vi "2 Channel Oscilloscope-iterate_filename.vi"() -> ()   [LabVIEW 2013]
doc: "The Two Channel Oscilloscope acquires and displays waveforms from one or two channels. Enter your Channel(s) and run the VI. While running, you can adjust the vertical position and volts per division, as well as the timebase. The Polarity can be set to get the best use of the range of your DAQ device. This VI supports digital and analog triggering. For digital triggering, you must connect the appropriate high-to-low or low-to-high TTL trigger signal to the trigger pin of your DAQ device. For analog trigger you set the trigger Level and Slope. View the help window description of each control for more information about its use."
panel:
  in  "input terminal configuration":i32(ring)=-1 items=["default"=-1, "RSE"=10083, "NRSE"=10078, "Differential"=10106, "Pseudodifferential"=12529]
  out "File Name Out Location":path caption="File Name Out"
  in  "Save to File":bool
  in  "digital source":tag="/Dev1/PFI0"
  in  "Trigger not recieved":string="Trigger Level is Out of Range or Trigger was not Recieved"
  in  "Channel B":tag="Dev1/ai1"
  in  "Channel A":tag="Dev1/ai0"
  in  "trigger support":string="Your hardware does not support this trigger mode."
  in  "invalid timebase":string="Invalid Timebase"
  out "Acquired":bool=TRUE
  in  "A/B switches":T1={"Position A"=-0.7490503006368473, "on/off A"=TRUE, "Position B"=-0.4188678921837484, "on/off B"=TRUE} {"Position B" min=-5.0 max=5.0 scale=-5.0..5.0 scale format="%0.1f"; "Position A" min=-5.0 max=5.0 scale=-5.0..5.0 scale format="%0.1f"}
  in  "Stop":bool
  in  "Timebase":u32(knob)=7 scale=0.0..11.0
  in  "Acquire On":bool=TRUE
  in  "Acquire Once":bool
  out "Timeout":bool
  in  "Slope":bool
  in  "Volts/Div B":u32(knob)=6 scale=0.0..9.0
  in  "Mode":u16(ring) items=["None", "Digital", "Hardware  Analog ", "Reference Analog"]
  in  "Position":i32(knob) min=0 max=497 scale=0.0..497.0
  in  "Level":dbl(knob)=0.5 min=-10.0 max=10.0 step=0.1 scale=-10.0..10.0
  in  "Channel":bool
  in  "Volts/Div A":u32(knob)=6 scale=0.0..9.0
  out "scope graph":sgl[][](graph)=[[-0.2881528, -0.23340708, -0.1802715, -0.12874603, -0.080118895, -0.032135844, 0.014237046, 0.054813385, 0.093135476, 0.12759316, 0.15850842, 0.182661, 0.2039153, 0.22001702, 0.23289835, 0.24320346, 0.24867809, 0.2538306, 0.2551188, 0.2586611, 0.25801712, 0.25544077, 0.25254244, 0.24738991, 0.23805094, 0.22420347, 0.2077797, 0.18813556, 0.16011858, 0.12888128, 0.093779504, 0.054169297, 0.011982858, -0.032779932, -0.081729114, -0.13228846, -0.18284774, -0.2366274, -0.2916952, -0.3451528, -0.40215275, -0.45689845, -0.5122882, -0.56864405, -0.6214576, -0.67620325, -0.72772855, -0.7821522, -0.83206725, -0.87844, -0.9248128, -0.96796525, -1.0091854, -1.043643, -1.0764903, -1.1070834, -1.1305919, -1.1476595, -1.162151, -1.1734221, -1.1850153, -1.1885576, -1.1917781, -1.1940322, -1.1972525, -1.1991848, -1.1943543, -1.1888797, -1.1834052, -1.1740662, -1.1573205, -1.1389647, -1.1164224, -1.0900156, -1.0545921, -1.0194905, -0.9795584, -0.936084, -0.8903552, -0.839152, -0.7895589, -0.7399658, -0.6852201, -0.6304745, -0.5754068, -0.519695, -0.46527132, -0.4076273, -0.3528816, -0.29749182, -0.24467826, -0.19057655, -0.13905114, -0.089135885, -0.04083079, 0.0026438236, 0.048050642, 0.08637273, 0.12018633, 0.15110165, 0.17879659, 0.1994068, 0.21615261, 0.22838992, 0.23837298, 0.24771196, 0.25157636, 0.25318652, 0.25576288, 0.25769502, 0.25737303, 0.25189847, 0.2461018, 0.23644078, 0.22549158, 0.20874578, 0.18716949, 0.16301692, 0.13338977, 0.09893209, 0.05835575, 0.017457426, -0.027627349, -0.0759325, -0.12649184, -0.17801726, -0.22922063, -0.28525454, -0.34257653, -0.39700022, -0.45013577, -0.50745773, -0.5641356, -0.6198474, -0.6749151, -0.7267624, -0.7789318, -0.83077914, -0.8797282, -0.92513484, -0.9695754, -1.0120838, -1.0484735, -1.0800326, -1.1093377, -1.1351002, -1.1560323, -1.1734221, -1.1834052, -1.1921, -1.201117, -1.2046593, -1.2053034, -1.2085238, -1.2101339, -1.2085238, -1.2024051, -1.1943543, -1.1859814, -1.1750324, -1.1550663, -1.132846, -1.1057953, -1.0745581, -1.0391345, -0.99855834, -0.95605, -0.9122535, -0.86298245, -0.8127453, -0.75799966, -0.7067964, -0.6530168, -0.596983, -0.5406272, -0.48427132, -0.43049172, -0.37574598, -0.31874603, -0.26367825, -0.21054268, -0.15901726, -0.10684776, -0.058220625, -0.014423966, 0.030982852, 0.071881175, 0.10794902, 0.14015245, 0.16784745, 0.19006783, 0.20745766, 0.22420347, 0.23225433, 0.24094927, 0.24738991, 0.24867809, 0.25125438, 0.26188153, 0.25415272, 0.25093234, 0.24481368, 0.23579669, 0.22645772, 0.21164411, 0.19167799, 0.16688132, 0.13822025, 0.10505074, 0.06801677, 0.02518624, -0.020220578, -0.067237556, -0.116830826, -0.16835624, -0.22181386, -0.27527148, -0.32937315, -0.385407, -0.4420849, -0.49876282, -0.55222034, -0.6072881, -0.66396594, -0.7180675, -0.7689488, -0.82079613, -0.86974514, -0.91869414, -0.9618466, -1.0027448, -1.0426768, -1.0774564, -1.1077275, -1.1318799, -1.1534561, -1.1695578, -1.1843712, -1.191134, -1.2001508, -1.2065915, -1.2088457, -1.2078797, -1.2082016, -1.2078797, -1.2062695, -1.2007949, -1.1895238, -1.1769645, -1.1615069, -1.1396087, -1.1122359, -1.0826089, -1.0491176, -1.0104735, -0.96667707, -0.92030436, -0.8726435, -0.8256266, -0.77313524, -0.71903366, -0.66396594, -0.6108304, -0.5535085, -0.49876282, -0.44240695, -0.38701716, -0.33227146, -0.27752572, -0.22245795, -0.1699664, -0.12101722, -0.06916976, -0.022474825, 0.01938963, 0.060609996, 0.09732193, 0.1321016, 0.16011858, 0.182661, 0.20262712, 0.21840686, 0.2312882, 0.2377289, 0.24449164, 0.24738991, 0.25125438, 0.25286454, 0.25318652, 0.2499662, 0.24642384, 0.23869503, 0.22838992, 0.21357632, 0.19683051, 0.17235589, 0.14466095, 0.111813426, 0.07703376, 0.03581339, -0.007983267, -0.055966377, -0.10394943, -0.15450877, -0.20539016, -0.26239014, -0.31649178, -0.3709155, -0.42694935, -0.48427132, -0.53966105, -0.59408474, -0.64947444, -0.70260996, -0.75799966, -0.80952495, -0.85718584, -0.9042027, -0.9525076, -0.99469393, -1.0323718, -1.0671513, -1.1006428, -1.1273715, -1.1489477, -1.1647272, -1.1798629, -1.1921, -1.1988628, -1.2024051, -1.2059474, -1.2130322, -1.210778, -1.2082016, -1.2078797, -1.2030492, -1.1959645, -1.181795, -1.1634392, -1.1457274, -1.122219, -1.0909817, -1.0558802, -1.0188464, -0.97988045, -0.93447375, -0.88552475, -0.83593166, -0.78569454, -0.73288107, -0.6778134, -0.62177956, -0.56864405, -0.5116441, -0.4552883, -0.39893243, -0.3441867, -0.29040706, -0.2346952, -0.18155962, -0.13035625, -0.081729114, -0.032779932, 0.011982858, 0.054169297, 0.0899151, 0.12437278, 0.15367794, 0.17944068, 0.19876271, 0.21583056, 0.22774583, 0.2370848, 0.24320346, 0.24706793, 0.25028825, 0.25189847, 0.25222045, 0.25028825, 0.24738991, 0.24030519, 0.23096615, 0.21776277, 0.1994068, 0.17879659, 0.15238976, 0.1195423, 0.08444053, 0.044830322, 0.0010336637, -0.045017183, -0.09461045, -0.14388168, -0.19637316, -0.24983081, -0.3061867, -0.36028838, -0.41374597, -0.471712, -0.52838993, -0.5824915, -0.6391694, -0.6913388, -0.74640644, -0.7982538, -0.84913504, -0.8955078, -0.94091445, -0.9863211, -1.025287, -1.0591005, -1.0916258, -1.1206088, -1.1454053, -1.1653713, -1.1769645, -1.1888797, -1.1991848, -1.2043374, -1.2069136, -1.2075577, -1.2127101, -1.2127101, -1.2072356, -1.201439, -1.1927441, -1.1850153, -1.1698798, -1.1492697, -1.1254393, -1.0987105, -1.0658633, -1.0256091, -0.985033, -0.94284666, -0.8967959, -0.8455927, -0.7953555, -0.7425421, -0.6903727, -0.6340169, -0.5786271, -0.52323735, -0.46881372, -0.41181377, -0.3548138, -0.29974604, -0.2475766, -0.1928308, -0.1406613, -0.090424, -0.04405111, 0.0019997954, 0.046762526, 0.08444053, 0.11922026, 0.14916945, 0.1762203, 0.19811869, 0.21389836, 0.22710174, 0.2370848, 0.24481368, 0.24835604, 0.25093234, 0.2544747, 0.25576288, 0.25479668, 0.25157636, 0.24384755, 0.23547465, 0.22388142, 0.2077797, 0.18620336, 0.16108471, 0.13145757, 0.09571171, 0.056423545, 0.01455909, -0.028915524, -0.07883078, -0.12681383, -0.18188167, -0.23437315, -0.2887969, -0.34354264, -0.40022054, -0.45657644, -0.5110001, -0.5657458, -0.62242365, -0.67652524, -0.7293387, -0.7815081, -0.83206725, -0.8826265, -0.926745, -0.97118556, -1.0107956, -1.0500836, -1.0813208, -1.1109478, -1.1331681, -1.1569985, -1.1737442, -1.1824391, -1.191456, -1.1988628, -1.2036933, -1.2040153, -1.2053034, -1.2056254, -1.2053034, -1.200473, -1.1908119, -1.182117, -1.1695578, -1.152168, -1.1280155, -1.0996766, -1.0700496, -1.034626, -0.99179566, -0.94896525, -0.9035586, -0.8565418, -0.8053385, -0.75220305, -0.6984235, -0.645288, -0.5905423, -0.53193223, -0.4765425, -0.42340696, -0.366085, -0.31037316, -0.25466132, -0.20023757, -0.15128845, -0.09911895, -0.049847722, -0.0047629476, 0.03742355, 0.07896596, 0.11406767, 0.14562708, 0.17074573, 0.19586444, 0.21389836, 0.22710174, 0.23805094, 0.2441696, 0.25157636, 0.25350863, 0.25640684, 0.25769502, 0.2551188, 0.25318652, 0.24900013, 0.23869503, 0.22838992, 0.21357632, 0.19264406, 0.16816944, 0.13822025, 0.10569477, 0.067050695, 0.026152313, -0.019254506, -0.06498331, -0.11522061, -0.16771215, -0.22084779, -0.27559352, -0.32969517, -0.38572904, -0.4420849, -0.4977967, -0.55189836, -0.6076101, -0.66203374, -0.7183896, -0.76927084, -0.81983, -0.8691011, -0.91643995, -0.96281266, -1.0021007, -1.0394565, -1.0748801, -1.1057953, -1.1305919, -1.1508799, -1.1669815, -1.1830832, -1.1908119, -1.1969305, -1.201117, -1.2069136, -1.2088457, -1.2056254, -1.2056254, -1.2043374, -1.1966085, -1.1875916, -1.1727781, -1.1576426, -1.1370325, -1.1090156, -1.0771344, -1.0429989, -1.0062871, -0.9637788, -0.9180501, -0.86974514, -0.819186, -0.76862675, -0.71452516, -0.6607456, -0.6072881, -0.5525424, -0.4945764, -0.43822053, -0.38025448, -0.3271189, -0.27301723, -0.21794945, -0.16577995, -0.114254534, -0.06530535, -0.019898534, 0.024542153, 0.06479645, 0.101186335, 0.1340338, 0.16140676, 0.18684745, 0.2039153, 0.21679664, 0.23193228, 0.23837298, 0.24481368, 0.248034, 0.25028825, 0.25189847, 0.25189847, 0.24835604, 0.24577975, 0.23611873, 0.22581363, 0.21003395, 0.19264406, 0.16849148, 0.13983041, 0.10827106, 0.070271015, 0.030982852, -0.012491763, -0.06015283, -0.11006808, -0.16062742, -0.213763, -0.26722065, -0.32357654, -0.37800023, -0.43339002, -0.4897459, -0.54545766, -0.6027796, -0.65655917, -0.71066076, -0.7650844, -0.8166097, -0.8639486, -0.9116094, -0.9583042, -1.0001686, -1.0375243, -1.072948, -1.103219, -1.1322019, -1.1534561, -1.1695578, -1.1840492, -1.1953204, -1.2053034, -1.2069136, -1.2111, -1.2146423, -1.2143203, -1.2123882, -1.2082016, -1.2020831, -1.1978967, -1.1837273, -1.1673036, -1.1450833, -1.122863, -1.092592, -1.0581344, -1.0191684, -0.97730416, -0.9328636, -0.8845587, -0.83593166, -0.78247416, -0.732559, -0.6771693, -0.6208135, -0.5657458, -0.51132214, -0.45593235, -0.39700022, -0.34193245, -0.28750876, -0.23340708, -0.1802715, -0.12906808, -0.08044094, -0.033746004, 0.010694683, 0.054169297, 0.091525316, 0.12533891, 0.1533559, 0.17847455, 0.19844067, 0.21325427, 0.22613567, 0.23418653, 0.2415933, 0.2441696, 0.24771196, 0.24932212, 0.24900013, 0.24674588, 0.24288148, 0.2370848, 0.22613567, 0.21357632, 0.19457626, 0.17299998, 0.14627111, 0.115033805, 0.078321874, 0.038389623, -0.0037968159, -0.04952568, -0.09815282, -0.15257657, -0.20216978, -0.25594944, -0.3100511, -0.3683392, -0.42308494, -0.4765425, -0.53354245, -0.5898983, -0.645288, -0.69681334, -0.7505929, -0.80276227, -0.85428756, -0.90066034, -0.9454229, -0.9888973, -1.0291514, -1.0661852, -1.0967784, -1.1238291, -1.1479816, -1.1676255, -1.1792188, -1.191134, -1.201761, -1.2072356, -1.2075577, -1.2123882, -1.2352524, -1.2143203, -1.210778, -1.2046593, -1.1946763, -1.1869476, -1.1705239, -1.1508799, -1.1260834, -1.0990326, -1.0652192, -1.0256091, -0.985355, -0.9399483, -0.8955078, -0.8462367, -0.79310125, -0.7406099, -0.68876255, -0.6327287, -0.57572883, -0.520017, -0.4649493, -0.40859342, -0.35159346, -0.29716977, -0.24403417, -0.19057655, -0.1387291, -0.08784777, -0.0382545, 0.005542159, 0.04708457, 0.08540666, 0.121474504, 0.15013552, 0.17654234, 0.20005089, 0.21486443, 0.22742379, 0.23805094, 0.24577975, 0.24932212, 0.25254244, 0.2538306, 0.2538306, 0.25125438, 0.24900013, 0.24288148, 0.23354244, 0.22259331, 0.20552546, 0.18201697, 0.15786433, 0.12823719, 0.092169344, 0.052237093, 0.0097286105, -0.035678208, -0.08462739, -0.13293248, -0.18703419, -0.23984778, -0.29330537, -0.3480511, -0.404729, -0.46237305, -0.51550853, -0.57250845, -0.6272541, -0.68360996, -0.73545736, -0.7866606, -0.83721983, -0.8868129, -0.9335077, -0.97537196, -1.0165921, -1.05427, -1.0871174, -1.1132021, -1.1386427, -1.1573205, -1.1753544, -1.1869476, -1.1937102, -1.2001508, -1.2053034, -1.2085238, -1.2091677, -1.2088457, -1.2098119, -1.2049813, -1.1949984, -1.1843712, -1.1708459, -1.1541002, -1.1280155, -1.1012869, -1.0690836, -1.0349481, -0.995016, -0.94960934, -0.9022705, -0.8546096, -0.8046945, -0.751881, -0.6984235, -0.6443219, -0.5905423, -0.53193223, -0.4775086, -0.42018664, -0.3683392, -0.31101722, -0.25498334, -0.20184779, -0.15000027, -0.10008502, -0.050813794, -0.0054070354, 0.03581339, 0.076711714, 0.112457514, 0.14305079, 0.17138982, 0.19200003, 0.21003395, 0.22291529, 0.23386449, 0.23998314, 0.24545771, 0.24932212, 0.25093234, 0.25350863, 0.25093234, 0.248034, 0.2441696, 0.23547465, 0.22259331, 0.20713562, 0.18813556, 0.16237283, 0.13145757, 0.099576116, 0.06093204, 0.018101454, -0.027949393, -0.07496637, -0.1242376, -0.17544097, -0.22954267, -0.28428844, -0.33774602, -0.39281377, -0.45077983, -0.5071357, -0.56381357, -0.615983, -0.6720168, -0.72579634, -0.7798979, -0.8275588, -0.87682986, -0.9248128, -0.9698974, -1.0101515, -1.0465412, -1.0787445, -1.1122359, -1.1370325, -1.1553884, -1.172134, -1.1872696, -1.1978967, -1.2027271, -1.2062695, -1.2117441, -1.2133542, -1.2091677, -1.2111, -1.2065915, -1.1998289, -1.1901679, -1.1769645, -1.1592528, -1.1367104, -1.1112698, -1.0784225, -1.0423548, -1.004999, -0.96410084, -0.91515183, -0.86684686, -0.81725377, -0.7670166, -0.71194893, -0.6575253, -0.6027796, -0.549, -0.4929662, -0.43435612, -0.37896633, -0.3242206, -0.26915282, -0.21472913, -0.16288167, -0.11296642, -0.064017236, -0.015068054, 0.0267964, 0.06737274, 0.10344058, 0.13725418, 0.16527116, 0.18684745, 0.20455933, 0.21969497, 0.23289835, 0.23933905, 0.24481368, 0.24738991], [-0.12800416, -0.1273601, -0.12703806, -0.12800416, -0.12800416, -0.126394, -0.12671602, -0.12703806, -0.12703806, -0.12607196, -0.12574992, -0.126394, -0.12671602, -0.1273601, -0.12607196, -0.1254279, -0.126394, -0.126394, -0.1254279, 1.4750845, 4.1615305, 4.1624966, 4.1541233, 4.1557336, 4.157022, 4.1615305, 4.153157, 4.1544456, 4.156378, 4.1605644, 4.1618524, 4.1541233, 4.15509, 4.160242, 4.1612086, 4.1538014, 4.1554117, 4.157022, 4.1618524, 4.1457505, 4.1541233, 4.157022, 4.1628184, 4.164107, 4.1554117, 4.1576657, 4.164107, 4.164107, 4.1557336, 4.15831, 4.1673274, 4.166361, 4.1518693, 4.160242, 4.1618524, 4.1676493, 4.1699038, 4.160242, 4.1621747, 4.168937, 4.168937, 4.1586323, 4.1615305, 4.1695814, -0.118343145, -0.118343145, -0.11963129, -0.120919436, -0.12188554, -0.12188554, -0.121563494, -0.12188554, -0.122529596, -0.12285164, -0.12285164, -0.12220755, -0.124139756, -0.1234957, -0.12220755, -0.123173654, -0.1234957, -0.1244618, -0.1234957, -0.1234957, -0.12381774, -0.124783844, -0.1254279, -0.1244618, -0.124139756, -0.1254279, -0.1254279, -0.1244618, -0.124783844, -0.12510586, -0.12574992, -0.1254279, -0.12510586, -0.1254279, -0.12703806, -0.126394, -0.126394, -0.12607196, -0.1273601, -0.12703806, -0.126394, -0.1273601, -0.12800416, -0.12768212, -0.1273601, 4.1576657, 4.1586323, 4.1621747, 4.163141, 4.156378, 4.157022, 4.1618524, 4.1624966, 4.15509, 4.156056, 4.1612086, 4.1612086, 4.151547, 4.1547675, 4.15509, 4.1595984, 4.157988, 4.1528354, 4.1538014, 4.159276, 4.1595984, 4.151225, 4.1525135, 4.1586323, 4.159276, 4.149937, 4.1518693, 4.1534796, 4.15992, 4.143174, 4.152191, 4.1538014, 4.15992, 4.1605644, 4.151225, 4.1528354, 4.159276, 4.160242, 4.149937, 4.151547, 4.1586323, 4.1595984, 4.1418858, 4.149937, -0.14571601, -0.12929231, -0.13122451, -0.12993637, -0.13090247, -0.13219061, -0.13219061, -0.13219061, -0.13251263, -0.13347873, -0.13283467, -0.13186857, -0.13251263, -0.13251263, -0.13347873, -0.13380077, -0.13283467, -0.13315669, -0.13347873, -0.13380077, -0.13283467, -0.13283467, -0.13315669, -0.13315669, -0.13219061, -0.13186857, -0.13186857, -0.13315669, -0.13283467, -0.13186857, -0.13186857, -0.13251263, -0.13251263, -0.13186857, -0.13186857, -0.13219061, -0.13219061, -0.13122451, -0.13122451, -0.13154653, -0.13219061, -0.13154653, -0.13122451, -0.13154653, -0.13219061, 4.1605644, 4.1541233, 4.1557336, 4.160242, 4.1605644, 4.1541233, 4.1547675, 4.1612086, 4.1605644, 4.1476827, 4.1534796, 4.1547675, 4.15992, 4.1605644, 4.152191, 4.1538014, 4.158954, 4.1595984, 4.151547, 4.1528354, 4.160242, 4.158954, 4.147361, 4.151547, 4.153157, 4.15831, 4.15831, 4.150259, 4.1528354, 4.15831, 4.159276, 4.1489706, 4.150903, 4.1586323, 4.158954, 4.147361, 4.150581, 4.153157, 4.159276, 4.151547, 4.150259, 4.153157, 4.1595984, 4.1605644, 4.150903, -0.12929231, -0.13122451, -0.13219061, -0.13122451, -0.13219061, -0.13251263, -0.13315669, -0.13219061, -0.13251263, -0.13219061, -0.13315669, -0.13347873, -0.13251263, -0.13251263, -0.13380077, -0.13347873, -0.13251263, -0.13219061, -0.13315669, -0.13412279, -0.13283467, -0.13219061, -0.13283467, -0.13347873, -0.13347873, -0.13283467, -0.13251263, -0.13315669, -0.13347873, -0.13251263, -0.13315669, -0.13347873, -0.13347873, -0.13219061, -0.13283467, -0.13283467, -0.13347873, -0.13315669, -0.13251263, -0.13283467, -0.13283467, -0.13315669, -0.13186857, -0.13219061, 4.1605644, 4.15831, 4.151225, 4.1538014, 4.1554117, 4.160242, 4.149937, 4.1534796, 4.1557336, 4.160242, 4.1608863, 4.1538014, 4.1554117, 4.1608863, 4.1615305, 4.153157, 4.15509, 4.159276, 4.1628184, 4.1463947, 4.1544456, 4.156056, 4.1634626, 4.163141, 4.1544456, 4.1557336, 4.1624966, 4.1628184, 4.1538014, 4.15509, 4.1624966, 4.1624966, 4.1480045, 4.1541233, 4.156056, 4.1621747, 4.1634626, 4.153157, 4.15509, 4.1615305, 4.1618524, 4.151547, 4.1534796, 4.1612086, 4.1612086, -0.12864822, -0.13058043, -0.13219061, -0.13315669, -0.13315669, -0.13219061, -0.13283467, -0.13380077, -0.13444483, -0.13283467, -0.13219061, -0.13380077, -0.13412279, -0.13283467, -0.13283467, -0.13380077, -0.13412279, -0.13347873, -0.13251263, -0.13283467, -0.13347873, -0.13315669, -0.13219061, -0.13251263, -0.13251263, -0.13315669, -0.13219061, -0.13219061, -0.13251263, -0.13251263, -0.13154653, -0.13154653, -0.13219061, -0.13251263, -0.13283467, -0.13122451, -0.13186857, -0.13251263, -0.13219061, -0.13122451, -0.13122451, -0.13219061, -0.13219061, -0.13122451, 4.1782765, 4.15509, 4.15992, 4.1608863, 4.1534796, 4.1544456, 4.15992, 4.1595984, 4.1528354, 4.1541233, 4.15992, 4.15992, 4.150903, 4.1538014, 4.1547675, 4.160242, 4.1586323, 4.152191, 4.1541233, 4.159276, 4.15992, 4.150259, 4.1525135, 4.159276, 4.159276, 4.149615, 4.151547, 4.153157, 4.159276, 4.142852, 4.151547, 4.152191, 4.157988, 4.1586323, 4.149615, 4.151547, 4.157344, 4.1586323, 4.149293, 4.150581, 4.15831, 4.157988, 4.142208, 4.150259, 4.151225, -0.12993637, -0.13186857, -0.13090247, -0.13154653, -0.13251263, -0.13315669, -0.13186857, -0.13251263, -0.13251263, -0.13283467, -0.13186857, -0.13219061, -0.13186857, -0.13283467, -0.13315669, -0.13186857, -0.13154653, -0.13219061, -0.13251263, -0.13154653, -0.13154653, -0.13219061, -0.13251263, -0.13122451, -0.13122451, -0.13154653, -0.13219061, -0.13154653, -0.13090247, -0.13090247, -0.13122451, -0.13122451, -0.13058043, -0.13025841, -0.13122451, -0.13122451, -0.12961432, -0.12993637, -0.13025841, -0.13058043, -0.12961432, -0.12897027, -0.12929231, -0.12993637, -0.13025841, 4.156056, 4.157988, 4.1634626, 4.1644287, 4.1566997, 4.158954, 4.165073, 4.165073, 4.1525135, 4.158954, 4.160242, 4.166039, 4.167005, 4.15831, 4.15992, 4.165717, 4.166039, 4.157988, 4.158954, 4.166039, 4.165717, 4.1534796, 4.15831, 4.1595984, 4.165717, 4.165395, 4.157022, 4.158954, 4.164751, 4.165395, 4.15509, 4.157344, 4.1644287, 4.1644287, 4.1528354, 4.156056, 4.1576657, 4.164107, 4.1538014, 4.156056, 4.157344, 4.1634626, 4.164751, 4.1557336, -0.13122451, -0.1273601, -0.1283262, -0.12800416, -0.12897027, -0.12897027, -0.12929231, -0.12864822, -0.12897027, -0.1283262, -0.12993637, -0.12993637, -0.12929231, -0.12864822, -0.13025841, -0.13025841, -0.12864822, -0.12897027, -0.12961432, -0.12993637, -0.12864822, -0.12929231, -0.12929231, -0.12929231, -0.12929231, -0.1283262, -0.12897027, -0.12897027, -0.12897027, -0.12800416, -0.12768212, -0.12864822, -0.12897027, -0.12768212, -0.1273601, -0.12800416, -0.12800416, -0.12864822, -0.1273601, -0.12768212, -0.1283262, -0.1283262, -0.1273601, -0.12768212, -0.12768212, 4.158954, 4.152191, 4.1541233, 4.1554117, 4.160242, 4.151225, 4.1534796, 4.1544456, 4.159276, 4.15992, 4.1518693, 4.153157, 4.158954, 4.159276, 4.151225, 4.1528354, 4.1547675, 4.160242, 4.1438184, 4.153157, 4.1547675, 4.160242, 4.1615305, 4.1525135, 4.1541233, 4.1595984, 4.1605644, 4.152191, 4.1538014, 4.1618524, 4.15992, 4.1457505, 4.1525135, 4.153157, 4.1586323, 4.159276, 4.150259, 4.152191, 4.1586323, 4.1586323, 4.1489706, 4.1518693, 4.1586323, 4.158954, 4.1460724, -0.12671602, -0.12897027, -0.13058043, -0.13122451, -0.13025841, -0.13090247, -0.13186857, -0.13283467, -0.13090247, -0.13154653, -0.13219061, -0.13283467, -0.13154653, -0.13154653, -0.13251263, -0.13283467, -0.13251263, -0.13186857, -0.13251263, -0.13283467, -0.13315669, -0.13186857, -0.13186857, -0.13315669, -0.13315669, -0.13219061, -0.13219061, -0.13283467, -0.13315669, -0.13186857, -0.13219061, -0.13219061, -0.13251263, -0.13315669, -0.13219061, -0.13219061, -0.13251263, -0.13347873, -0.13219061, -0.13251263, -0.13315669, -0.13283467, -0.13251263, -0.13251263, 4.1463947, 4.150259, 4.1518693, 4.144462, 4.1460724, 4.151225, 4.152191, 4.145428, 4.1470385, 4.1518693, 4.1525135, 4.14253, 4.145428, 4.1470385, 4.1518693, 4.151547, 4.145428, 4.1463947, 4.1525135, 4.1541233, 4.1447845, 4.1467166, 4.1534796, 4.1538014, 4.143496, 4.1463947, 4.1480045, 4.1528354, 4.1373773, 4.144462, 4.1467166, 4.1534796, 4.1538014, 4.1451063, 4.1463947, 4.1534796, 4.1541233, 4.144462, 4.1463947, 4.1557336, 4.1547675, 4.136733, 4.1457505, 4.1467166, 4.1541233, -0.13315669, -0.13380077, -0.13412279, -0.13541093, -0.13669908, -0.13573298, -0.13573298, -0.13669908, -0.13669908, -0.13573298, -0.136055, -0.13637704, -0.1370211, -0.13734314, -0.136055, -0.13637704, -0.13637704, -0.13766518, -0.13637704, -0.136055, -0.13637704, -0.1370211, -0.13573298, -0.136055, -0.13573298, -0.13669908, -0.13637704, -0.13573298, -0.136055, -0.136055, -0.13637704, -0.13541093, -0.13541093, -0.136055, -0.13637704, -0.13508889, -0.13541093, -0.136055, -0.13637704, -0.13541093, -0.13476688, -0.13508889, -0.13541093, -0.13637704, 4.1586323, 4.151225, 4.156056, 4.157344, 4.150259, 4.151225, 4.157022, 4.1566997, 4.144462, 4.150581, 4.1525135, 4.157988, 4.1576657, 4.150259, 4.1525135, 4.1576657, 4.1586323, 4.150581, 4.152191, 4.1586323, 4.159276, 4.1463947, 4.151225, 4.153157, 4.1586323, 4.158954, 4.149937, 4.1518693, 4.157988, 4.1586323, 4.1489706, 4.151547, 4.1595984, 4.160242, 4.1480045, 4.151225, 4.153157, 4.158954, 4.151225, 4.150259, 4.1518693, 4.15831, 4.15831, 4.1486487, 4.149937, -0.13219061, -0.13347873, -0.13283467, -0.13347873, -0.13444483, -0.13508889, -0.13444483, -0.13444483, -0.13444483, -0.13573298, -0.13508889, -0.13412279, -0.13444483, -0.13508889, -0.13541093, -0.13412279, -0.13380077, -0.13412279, -0.13412279, -0.13347873, -0.13283467, -0.13347873, -0.13347873, -0.13380077, -0.13186857, -0.13251263, -0.13283467, -0.13347873, -0.13219061, -0.13186857, -0.13219061, -0.13251263, -0.13122451, -0.13154653, -0.13122451, -0.13186857, -0.13154653, -0.13058043, -0.13058043, -0.13122451, -0.13154653, -0.13058043, -0.13025841, -0.13090247, -0.13090247, 4.15509, 4.157988, 4.158954, 4.164107, 4.1547675, 4.157022, 4.15831, 4.1634626, 4.1634626, 4.1554117, 4.156378, 4.1624966, 4.1628184, 4.1544456, 4.156378, 4.157988, 4.1624966, 4.1463947, 4.1544456, 4.1566997, 4.1618524, 4.163141, 4.1538014, 4.156378, 4.1624966, 4.1634626, 4.1541233, 4.1554117, 4.163141, 4.163141, 4.1486487, 4.15509, 4.1566997, 4.163141, 4.164107, 4.1541233, 4.1557336, 4.1618524, 4.163141, 4.1525135, 4.15509, 4.1621747, 4.1624966, 4.150903, -0.12929231, -0.12961432, -0.13090247, -0.13186857, -0.13122451, -0.13186857, -0.13251263, -0.13251263, -0.13154653, -0.13219061, -0.13315669, -0.13315669, -0.13154653, -0.13315669, -0.13315669, -0.13347873, -0.13251263, -0.13251263, -0.13251263, -0.13347873, -0.13347873, -0.13251263, -0.13219061, -0.13347873, -0.13347873, -0.13251263, -0.13251263, -0.13251263, -0.13283467, -0.13219061, -0.13219061, -0.13219061, -0.13283467, -0.13347873, -0.13186857, -0.13186857, -0.13283467, -0.13283467, -0.13186857, -0.13219061, -0.13219061, -0.13315669, -0.13219061, -0.13251263, -0.13251263, 4.1628184, 4.1634626, 4.156378, 4.1576657, 4.163141, 4.1628184, 4.156378, 4.157344, 4.163785, 4.1634626, 4.1538014, 4.156378, 4.1576657, 4.163141, 4.1612086, 4.1547675, 4.156378, 4.160242, 4.1605644, 4.151225, 4.153157, 4.158954, 4.1595984, 4.149937, 4.1525135, 4.153157, 4.1595984, 4.144462, 4.152191, 4.1528354, 4.158954, 4.1595984, 4.150259, 4.1518693, 4.15831, 4.1586323, 4.149615, 4.1518693, 4.1586323, 4.158954, 4.142852, 4.150903, 4.1528354, 4.159276, -0.17952953, -0.12961432, -0.13186857, -0.13315669, -0.13315669, -0.13315669, -0.13347873, -0.13444483, -0.13412279, -0.13347873, -0.13347873, -0.13315669, -0.13508889, -0.13412279, -0.13380077, -0.13347873, -0.13476688, -0.13508889, -0.13347873, -0.13380077, -0.13444483, -0.13476688, -0.13380077, -0.13315669, -0.13347873, -0.13380077, -0.13412279, -0.13283467, -0.13347873, -0.13380077, -0.13412279, -0.13283467, -0.13315669, -0.13315669, -0.13347873, -0.13283467, -0.13251263, -0.13315669, -0.13347873, -0.13251263, -0.13186857, -0.13251263, -0.13315669, -0.13315669]]
  # "/div"
  # "/div"
  # "TIMEBASE"
  # "TRIGGER"
  # "/div"
  # "CHANNEL A\nVERTICAL"
  # "CHANNEL B\nVERTICAL"
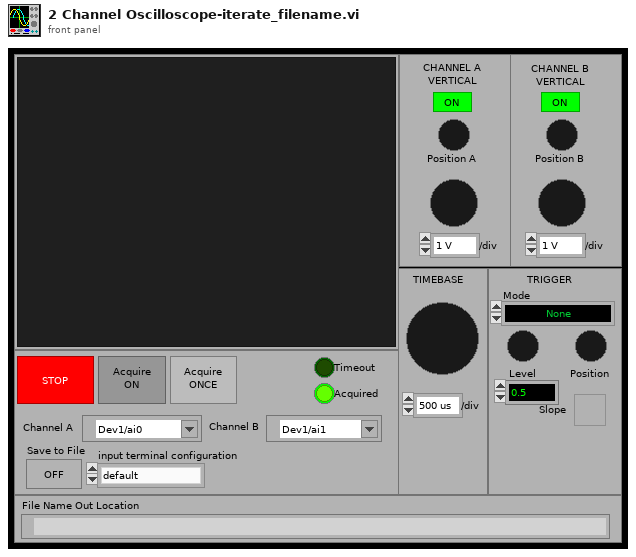
[diagram p1: front panel]
types:
  T1 = cluster{"Position A":dbl, "on/off A":bool, "Position B":dbl, "on/off B":bool}
  T2 = cluster{"Volts/Div A":u32, "Volts/Div B":u32, "Timebase":u32, "Polarity":bool, "input terminal configuration":i32}
  T3 = cluster{"Channel":bool, "Level":dbl, "Mode":u16, "Slope":bool, "Position":i32, "digital source":tag}
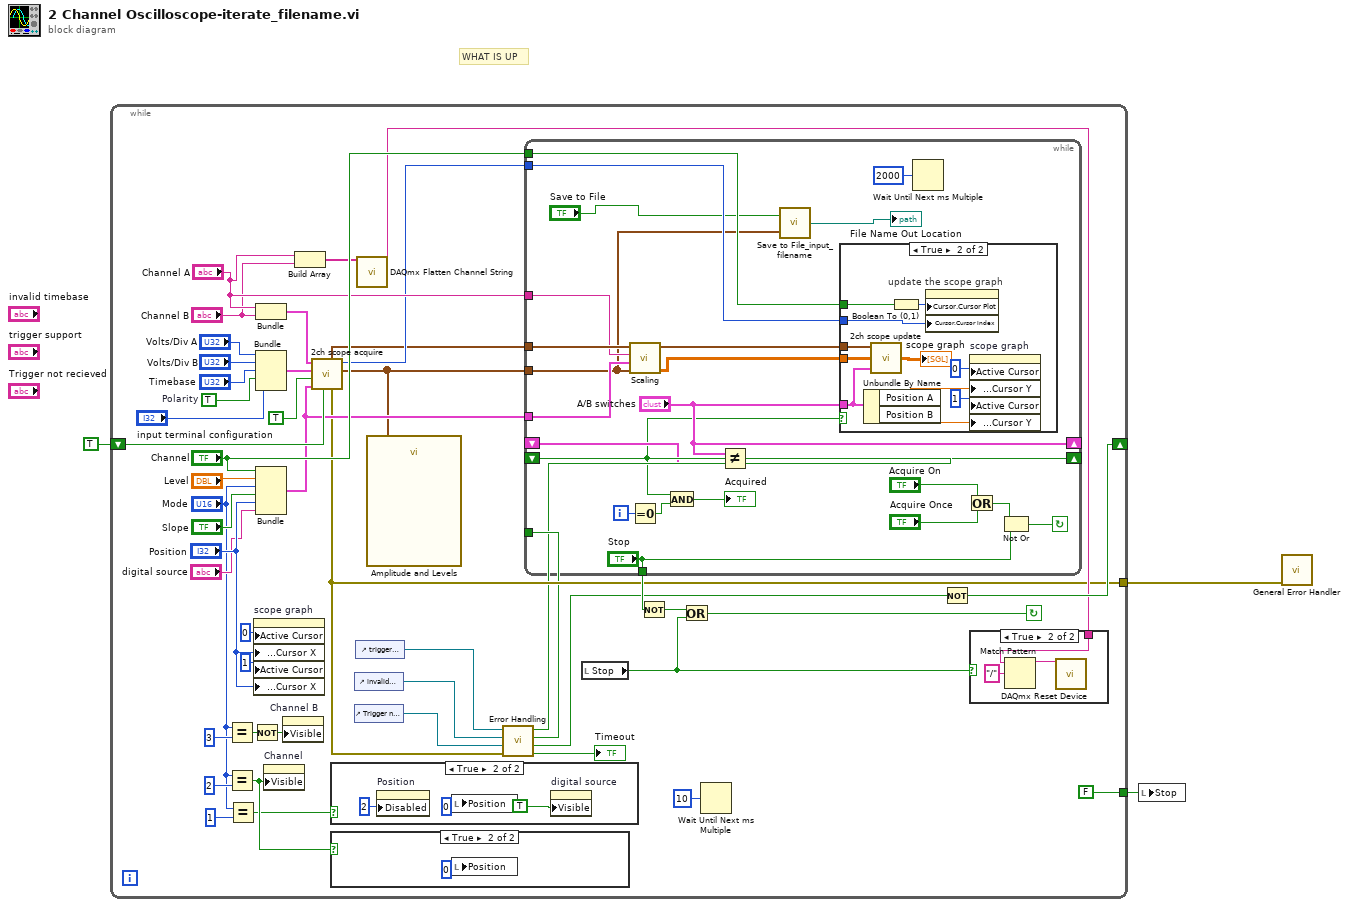
[diagram p0: block diagram]
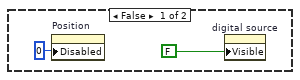
[diagram p2: hidden frame]
diagram:
  # "WHAT IS UP"
  n1 = while {
    shift-left: TRUE -> [w23]
    shift-right: [w40] -> _
    tunnel: [w15] -> w1
    tunnel: [FALSE] -> w2
    stop <- w28 continue-if-true
    w26 = TRUE  # Polarity
    n2 = Equal?(x="Mode", y=u16 3) -> (x = y?=w10:bool)
    n3 = Equal?(x="Mode", y=u16 2) -> (x = y?=w6:bool)
    n4 = Equal?(x="Mode", y=u16 1) -> (x = y?=w5:bool)
    n5 = Not(x=w10) -> (.not. x?=w9:bool)
    n6 = property on="scope graph" class="WFGraph (strict)"("Active Cursor"=u32 0, "Cursor.Cursor Position:Cursor X"="Position", "Active Cursor"=u32 1, "Cursor.Cursor Position:Cursor X"="Position") -> ()  [unwired: 2 in, 2 out]
    n7 = Bundle("Channel A"="Channel A", "Channel B"="Channel B") -> (w19:cluster{"Channel A":tag, "Channel B":tag})  [unwired: 1 out]
    n8 = Bundle("Volts/Div A"="Volts/Div A", "Volts/Div B"="Volts/Div B", "Timebase"="Timebase", "Polarity"=w26, "input terminal configuration"="input terminal configuration") -> (w20:T2)  [unwired: 1 out]
    n9 = Bundle("Channel"="Channel", "Level"="Level", "Mode"="Mode", "Slope"="Slope", "Position"="Position", "digital source"="digital source") -> (w22:T3)  [unwired: 1 out]
    n10 = property on="Channel" class="Bool (strict)"("Visible"=w6) -> ()  [unwired: 2 in, 2 out]
    n11 = property on="Channel B" class="DAQmxName"("Visible"=w9) -> ()  [unwired: 2 in, 2 out]
    n12 = Build Array("Channel A", "Channel B") -> (w32:tag[])
    n13 = call "2ch scope acquire.vi"("config?"=w23, "Trigger"=w22, "clear acquisition?"=TRUE, "volts/time"=w20, "Channels"=w19) -> ("data"=w4:waveform(dbl)[], "pretrigger position"=w25:i32, "error out"=w15:errorcluster, "Scaling"=w24:cluster{"volts/div A":sgl, "volts/div B":sgl})  [unwired: 3 out]
    n14 = case shown="True" w5 {
      frame False {
        n15 = property on="Position" class="Knob (strict)"("Disabled"=u8 0) -> ()  [unwired: 2 in, 2 out]
        n16 = property on="digital source" class="DAQmxName"("Visible"=FALSE) -> ()  [unwired: 2 in, 2 out]
      }
      frame True {
        n17 = property on="Position" class="Knob (strict)"("Disabled"=u8 2) -> ()  [unwired: 2 in, 2 out]
        n18 = local write "Position"(0 ("Position")) -> ()
        n19 = property on="digital source" class="DAQmxName"("Visible"=TRUE) -> ()  [unwired: 2 in, 2 out]
      }
    }
    n20 = case shown="True" w6 {
      frame False {
      }
      frame True {
        n21 = local write "Position"(0 ("Position")) -> ()
      }
    }
    n22 = control-ref of="invalid timebase"() -> (w17:refnum<vi>)
    n23 = control-ref of="Trigger not recieved"() -> (w16:refnum<vi>)
    n24 = control-ref of="trigger support"() -> (w18:refnum<vi>)
    n25 = call <vilib>:"DAQmx Flatten Channel String.vi"("names in"=w32) -> ("names out"=w29:string)  [unwired: 1 in, 13 out]
    n26 = call "Amplitude and Levels"("input signals"=w4) -> ()  [unwired: 16 in, 3 out]
    n27 = call "Error Handling.vi"("error out"=w15, "Str Refnum"=w16, "reference 2"=w17, "reference"=w18) -> ("Boolean"=→"Timeout":bool, "Boolean 2"=w13:bool, "Boolean 3"=w12:bool, "Boolean 4"=w11:bool)
    n28 = while {
      tunnel: w24 -> [w64]
      tunnel: w4 -> [w57]
      tunnel: w25 -> [w70]
      tunnel: "Channel" -> [w71]
      shift-left: w11 -> [w69]
      shift-right: [w76] -> _
      shift-left: _ -> [w74]
      shift-right: ["A/B switches"] -> _
      tunnel: ["Stop"] -> w41
      tunnel: w12 -> [_]
      tunnel: "Channel A" -> [w63]
      tunnel: w22 -> [w62]
      i -> [w73]
      stop <- w59 continue-if-true
      n29 = call "Scaling.vi"("data"=w57, "Cluster"=w62, "Channel A"=w63, "Scaling"=w64) -> ("voltage data"=w60:dbl[][], "Scaling 2"=w61:cluster{"volts/div A":sgl, "volts/div B":sgl})  [unwired: 2 out]
      n30 = Equal To 0?(x=w73) -> (x = 0?=w72:bool)
      n31 = And(x=w69, y=w72) -> (x .and. y?=→"Acquired":bool)
      n32 = Not Equal?(x="A/B switches", y=w74) -> (x != y?=w76:bool)
      n33 = call "Save to File_input_filename.vi"("data"=w57, "Save to File"="Save to File") -> ("File Name Out Location"=→"File Name Out Location":path)
      n34 = case shown="True" w69 {
        tunnel: w70 -> [_ w89]
        tunnel: w71 -> [_ w90]
        tunnel: "A/B switches" -> [_ w88]
        tunnel: w61 -> [_ w81]
        tunnel: w60 -> [_ w80]
        frame False {
          # "no user changes to front\npanel switches,so do not\nupdate the scope graph"
        }
        frame True {
          # "update the scope graph"
          n35 = Unbundle By Name(w88) -> ("Position A"=w85:dbl, "Position B"=w84:dbl)
          n36 = call "2ch scope update.vi"("A/B switches"=w88, "voltage data"=w80, "Scaling"=w81) -> ("scope graph"=→"scope graph":sgl[][])  [unwired: 1 in, 1 out]
          n37 = Boolean To (0,1)(Boolean=w90) -> (0, 1=w82:i16)
          n38 = property on="scope graph" class="WFGraph (strict)"("Cursor.Cursor Plot"=w82, "Cursor.Cursor Index"=w89) -> ()  [unwired: 2 in, 2 out]
          n39 = property on="scope graph" class="WFGraph (strict)"("Active Cursor"=u32 0, "Cursor.Cursor Position:Cursor Y"=w85, "Active Cursor"=u32 1, "Cursor.Cursor Position:Cursor Y"=w84) -> ()  [unwired: 2 in, 2 out]
        }
      }
      n40 = Wait Until Next ms Multiple(millisecond multiple=u32 2000) -> ()  [unwired: 1 out]
      n41 = Or(x="Acquire On", y="Acquire Once") -> (x .or. y?=w77:bool)
      n42 = Not Or(1:"Stop", 2:w77) -> (0:w59:bool)
    }
    n43 = local read "Stop"() -> (w31:bool)
    n44 = Not(x=w41) -> (.not. x?=w36:bool)
    n45 = Or(x=w36, y=w31) -> (x .or. y?=w28:bool)
    n46 = Wait Until Next ms Multiple(millisecond multiple=u32 10) -> ()  [unwired: 1 out]
    n47 = Not(x=w13) -> (.not. x?=w40:bool)
    n48 = case shown="True" w31 {
      tunnel: w29 -> [_ w91]
      frame False {
      }
      frame True {
        n49 = Match Pattern(string=w91, regular expression="/") -> (before substring=w92:string)  [unwired: 4 out]
        n50 = call <vilib>:"DAQmx Reset Device.vi"("device in"=w92) -> ()  [unwired: 1 in, 14 out]
      }
    }
  }
  n51 = local write "Stop"(w2) -> ()
  n52 = call <vilib>:"General Error Handler.vi"("error in (no error)"=w1) -> ()  [unwired: 1 in, 14 out]
